vi "Add Object Parameter - 1D Array String.vi"(8 "error in (no error)":errorcluster, 9 "Name":string, 10 "1D String":string[](array[string]), 11 "JSON Tree in (JSON Object)":variant) -> (0 "error out":errorcluster, 3 "JSON Tree out (JSON Object)":variant)   [LabVIEW 2015, in "i3-json.lvlib"]
doc: "Use this template to build a VI to use as a subVI."
uses:
  i3-json.lvlib
  JSON Types/JSON Type.ctl
  JSON Types/JSON Compatible Type.ctl
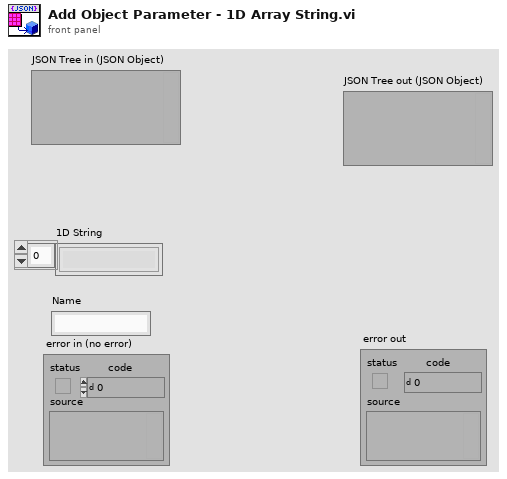
[diagram p1: front panel]
types:
  T1 = typedef "i3-json.lvlib/JSON Compatible Type.ctl" = enum16{"1D Double Array", "1D String Array", "1D Boolean Array", "Unknown"}
  T2 = typedef "i3-json.lvlib/JSON Type.ctl" = enum8{"JSON Compatible", "JSON Array", "JSON Object", "JSON Null", "Double", "String", "Boolean", "Unknown"}
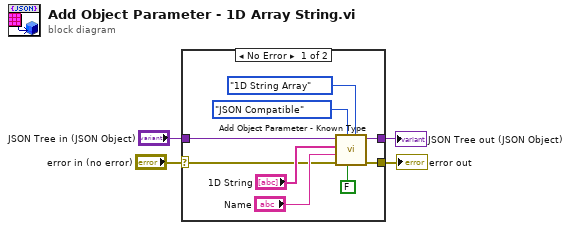
[diagram p0: block diagram]
diagram:
  n1 = case shown="No Error" "error in (no error)" {
    selector: "error in (no error)" -> [w5 w15]
    tunnel: [w13 w15] -> w3
    tunnel: [w12 w14] -> w2
    tunnel: "JSON Tree in (JSON Object)" -> [w11 w14]
    frame No Error {
      n2 = call "Add Object Parameter - Known Type.vi"("JSON Compatible Type"=JSON_Compatible_Type."1D String Array", "Add Parameter as JSON Tree?"=FALSE, "JSON Type"=JSON_Type."JSON Compatible", "error in (no error)"=w5, "Name"="Name", "Value"="1D String", "JSON Tree in (JSON Object)"=w11) -> ("error out"=w13:errorcluster, "JSON Tree out (JSON Object)"=w12:variant)  [unwired: 3 in]
    }
    frame Error {
    }
  }
  "error out" <- w3
  "JSON Tree out (JSON Object)" <- w2
